vi "Optical Encoder Counter 3.vi"(11 "Input":dbl) -> (3 "Output":dbl)   [LabVIEW 2020]
panel:
  in  "Last Value":bool
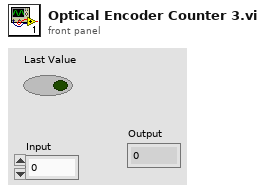
[diagram p1: front panel]
types:
  T1 = typedef "WPI_CounterDevRef.ctl" = cluster{"DevStatus":errorcluster, "CntIndex":T2}
  T2 = typedef "FPGA_CounterCtrSystemIndex.ctl" = enum8{"Ctr 0", "Ctr 1", "Ctr 2", "Ctr 3", "Ctr 4", "Ctr 5", "Ctr 6", "Ctr 7", "Invalid"}
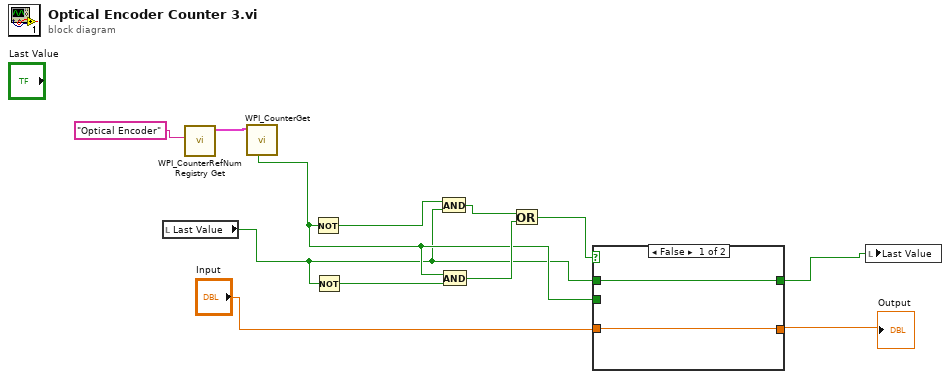
[diagram p0: block diagram]
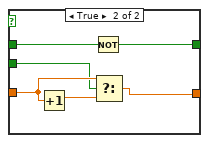
[diagram p2: hidden frame]
diagram:
  n1 = local read "Last Value"() -> (w3:bool)
  n2 = call <vilib>:"WPI_CounterRefNum Registry Get.vi"("refnum name"="Optical Encoder") -> ("CounterDevRef"=w11:T1)  [unwired: 9 in, 1 out]
  n3 = call <vilib>:"WPI_CounterGet.vi"("CounterDevRef in"=w11) -> ("Stopped"=w5:bool)  [unwired: 5 in, 5 out]
  n4 = Not(x=w5) -> (.not. x?=w6:bool)
  n5 = Not(x=w3) -> (.not. x?=w7:bool)
  n6 = And(x=w6, y=w3) -> (x .and. y?=w9:bool)
  n7 = And(x=w5, y=w7) -> (x .and. y?=w8:bool)
  n8 = Or(x=w9, y=w8) -> (x .or. y?=w10:bool)
  n9 = case shown="False" w10 {
    tunnel: "Input" -> [w13 w20]
    tunnel: w5 -> [_ w18]
    tunnel: [w13 w17] -> w2
    tunnel: w3 -> [w14 w16]
    tunnel: [w14 w15] -> w1
    frame False {
    }
    frame True {
      n10 = Increment(x=w20) -> (x+1=w19:dbl)
      n11 = Not(x=w16) -> (.not. x?=w15:bool)
      n12 = Select(t=w20, s=w18, f=w19) -> (s? t:f=w17:dbl)
    }
  }
  "Output" <- w2
  n13 = local write "Last Value"(w1) -> ()
